vi "writeFile.vi"() -> ()   [LabVIEW 2015]
panel:
  in  "file (use dialog)":path
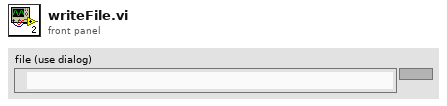
[diagram p1: front panel]
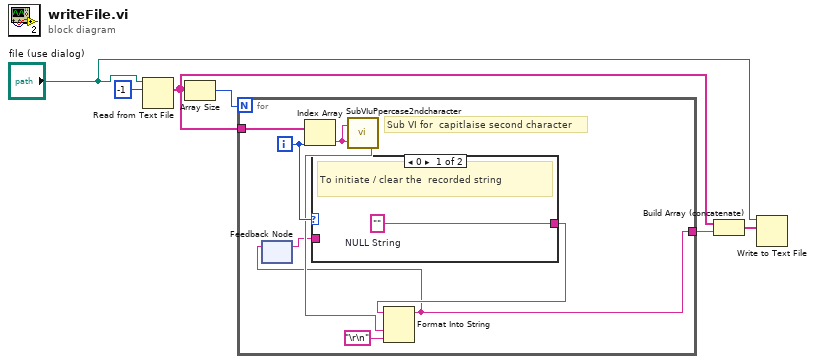
[diagram p0: block diagram]
diagram:
  n1 = Read from Text File(file (use dialog)="file (use dialog)", count=-1) -> (text=w3:string[])  [unwired: 2 in, 3 out]
  n2 = Array Size(array=w3) -> (size(s)=w5:i32)
  n3 = for {
    N: w5 -> [_]
    tunnel: w3 -> [w14]
    tunnel: [w7] -> w2
    i -> [w12]
    # "Sub VI for  capitlaise second character"
    n4 = feedback #1() -> (w8:string)  [unwired: 1 in]
    n5 = Index Array(array=w14, index=w12) -> (element=w13:string)
    n6 = case shown="0" w12 {
      tunnel: [w15 w16] -> w9
      tunnel: w8 -> [_ w16]
      frame 0 {
        w15 = ""  # NULL String
        # "To initiate / clear the  recorded string"
      }
      frame 1, Default {
        # "Work as normal feedback"
      }
    }
    n7 = call "SubVIuPpercase2ndcharacter.vi"("substring"=w13, "string"=w13) -> ("result string"=w11:string)
    n8 = Format Into String(initial string=w9, w11, "\r\n") -> (resulting string=w7:string)  [unwired: 2 in, 1 out]
    n9 = feedback-in #1(w7) -> ()
  }
  n10 = Build Array (concatenate)(w3, w2) -> (w1:string[])
  n11 = Write to Text File(file (use dialog)="file (use dialog)", text=w1) -> ()  [unwired: 2 in, 3 out]
